vi "twoAxiesControl_Example.vi"() -> ()   [LabVIEW 2020]
uses:
  Recipe.vi
  ConnectionData.vi
  ConnectionData_Write.vi
  SMCD14_lib.lvlib
panel:
  in  "StopAppBtn":bool caption="Close"
  in  "Recipe":bool
  in  "Chart":bool
  in  "DisconnectBtn":bool
  in  "ConnectBtn":bool
  out "AxisControlSubPanelsArray":refnum<vi>[](array[refnum])
  in  "error in (no error)":errorcluster
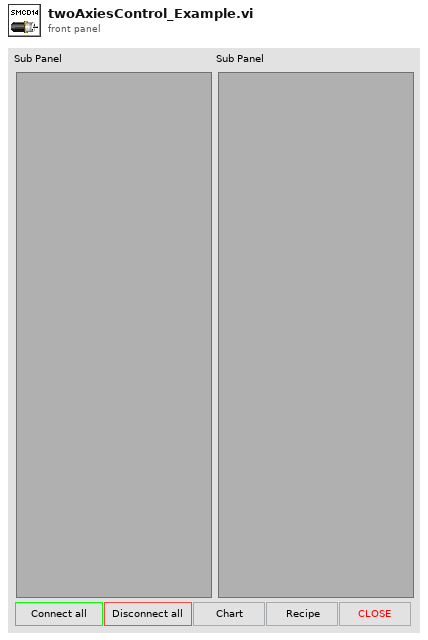
[diagram p1: front panel]
types:
  T1 = enum32{"Invalid", "Standard", "Closed", "Hidden", "Minimized", "Maximized"}
  T2 = enum32{"Bad", "Idle", "Run top level", "Running"}
  T3 = typedef "SMCD14_lib.lvlib/ConnectionData_typedef.ctl" = cluster{"DeviceIDCtrl":u16, "ProtocolCtrl":enum16{"Modbus RTU", "Modbus TCP", ""}, "COMportCtrl":refnum<visa-resource-name>, "IPCtrl":string, "serial master instance":refnum<class "Modbus Master.lvclass">, "ConnectionStatusIndicator":bool}
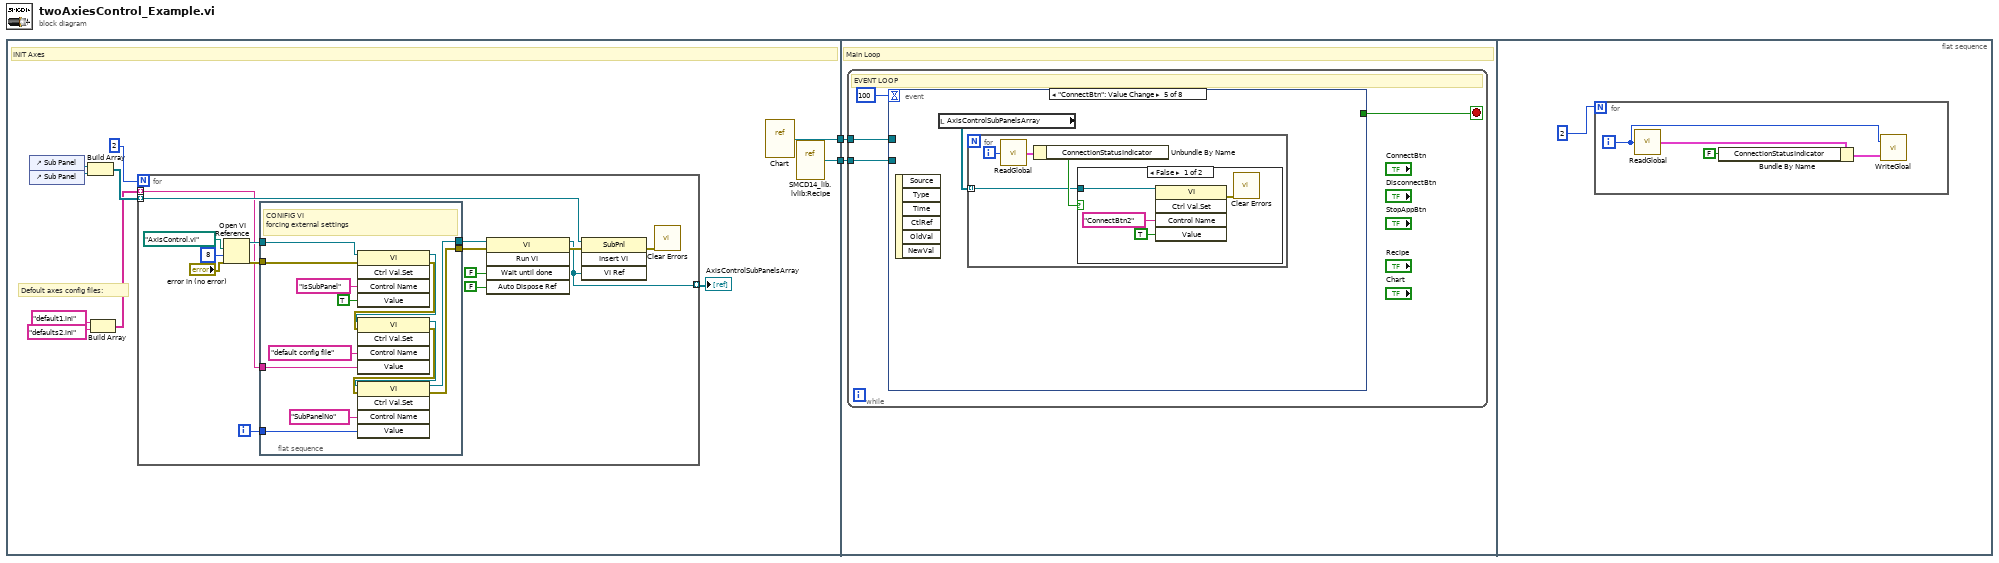
[diagram p0: block diagram]
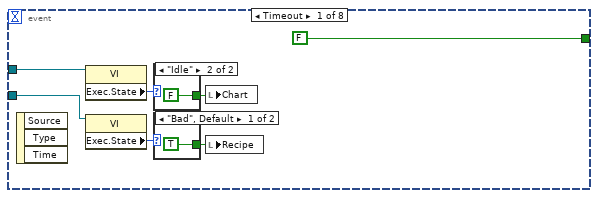
[diagram p2: hidden frame]
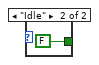
[diagram p3: hidden frame]
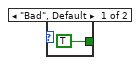
[diagram p4: hidden frame]
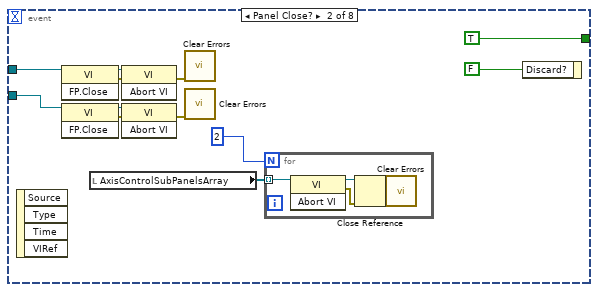
[diagram p5: hidden frame]
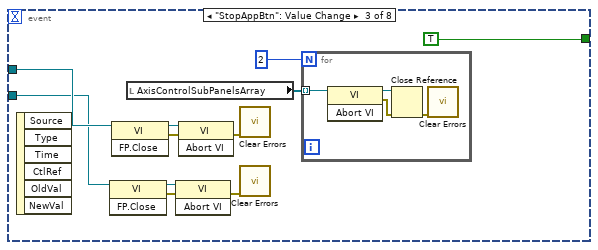
[diagram p6: hidden frame]
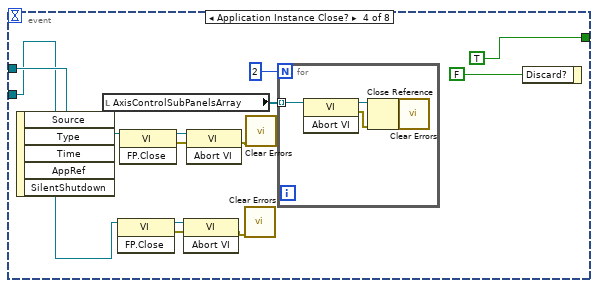
[diagram p7: hidden frame]
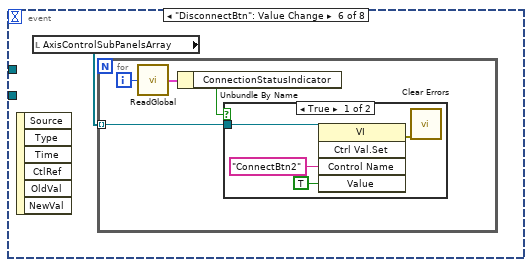
[diagram p9: hidden frame]
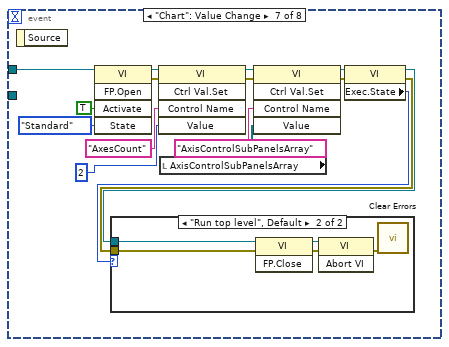
[diagram p11: hidden frame]
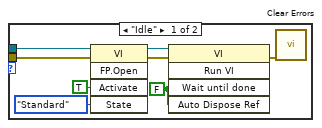
[diagram p12: hidden frame]
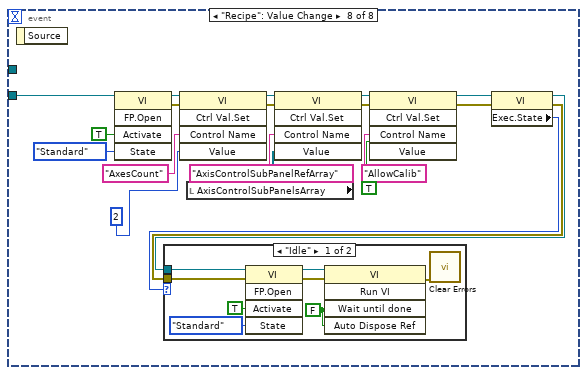
[diagram p13: hidden frame]
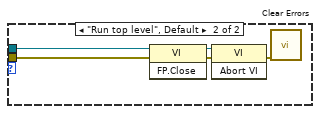
[diagram p14: hidden frame]
diagram:
  n1 = flat-sequence {
    tunnel: [w10] -> w2
    tunnel: [w9] -> w1
    tunnel: w2 -> [w43]
    tunnel: w1 -> [w42]
    frame #0 {
      # "Defoult axes config files:"
      # "INIT Axes"
      n2 = control-ref of="Sub Panel"() -> (w8:refnum<vi>)
      n3 = control-ref of="Sub Panel"() -> (w7:refnum<vi>)
      n4 = Build Array(w8, w7) -> (w11:refnum<vi>[])
      n5 = Build Array("default1.ini" ("default value"), "defaults2.ini" ("default value")) -> (w3:string[])
      n6 = for {
        N: 2 ("AxesCount") -> [_]
        tunnel: w11 -> [w24] mode=indexing
        tunnel: [w14] -> w12 mode=indexing
        tunnel: w3 -> [w16] mode=indexing
        i -> [w15]
        n7 = Open VI Reference(vi path=path "AxisControl.vi", options=8, error in (no error)="error in (no error)") -> (vi reference=w18:refnum<vi>, error out=w17:errorcluster)  [unwired: 3 in]
        n8 = flat-sequence {
          tunnel: w18 -> [w39]
          tunnel: [w30] -> w25
          tunnel: w17 -> [w38]
          tunnel: [w31] -> w23
          tunnel: w16 -> [w34]
          tunnel: w15 -> [w33]
          frame #0 {
            # "CONIFIG VI\nforcing external settings"
            n9 = invoke class="VI" method="Ctrl Val.Set"(reference=w39, error in=w38, "Control Name"="IsSubPanel", "Value"=TRUE) -> (reference out=w36:refnum<vi>, error out=w35:errorcluster)  [unwired: 1 in, 3 out]
            n10 = invoke class="VI" method="Ctrl Val.Set"(reference=w36, error in=w35, "Control Name"="default config file", "Value"=w34) -> (reference out=w29:refnum<vi>, error out=w28:errorcluster)  [unwired: 1 in, 3 out]
            n11 = invoke class="VI" method="Ctrl Val.Set"(reference=w29, error in=w28, "Control Name"="SubPanelNo", "Value"=w33) -> (reference out=w31:refnum<vi>, error out=w30:errorcluster)  [unwired: 1 in, 3 out]
          }
        }
        n12 = invoke class="VI" method="Run VI"(reference=w23, error in=w25, "Wait until done"=FALSE ("Wait Until Done"), "Auto Dispose Ref"=FALSE ("Auto Dispose Reference")) -> (reference out=w14:refnum<vi>, error out=w22:errorcluster)  [unwired: 1 in, 3 out]
        n13 = invoke class="SubPnl" method="Insert VI"(reference=w24, error in=w22, "VI Ref"=w14) -> (error out=w13:errorcluster)  [unwired: 1 in, 3 out]
        n14 = call <vilib>:"Clear Errors.vi"("error in (no error)"=w13) -> ()  [unwired: 5 in, 2 out]
      }
      "AxisControlSubPanelsArray" <- w12
      n15 = vi-ref "Chart.vi"() -> (w10:refnum<vi>)
      n16 = vi-ref "SMCD14_lib.lvlib:Recipe.vi"() -> (w9:refnum<vi>)
    }
    frame #1 {
      # "Main Loop"
      n17 = while {
        tunnel: w43 -> [w45]
        tunnel: w42 -> [w44]
        stop <- w46 stop-if-true
        # "EVENT LOOP"
        n18 = event shown="[4] \"ConnectBtn\": Value Change" {
          selector: _ -> [_ _ _ _ _ _ _ _]
          dyn-events: _ -> [_ _ _ _ _ _ _ _]
          timeout: 100 -> [_ _ _ _ _ _ _ _]
          tunnel: [FALSE ("Discard?") TRUE ("Discard?") TRUE ("Discard?") TRUE ("Discard?") _ _ _ _] -> w46
          tunnel: w45 -> [w53 w67 w83 w94 _ _ w134 _]
          tunnel: w44 -> [w49 w64 w80 w93 _ _ _ w161]
          event Timeout {
            n19 = event-data() -> ()  [unwired: 1 in, 3 out]
            n20 = property class="VI"(reference=w53) -> ("Exec.State"=w52:T2)  [unwired: 1 in, 2 out]
            n21 = property class="VI"(reference=w49) -> ("Exec.State"=w50:T2)  [unwired: 1 in, 2 out]
            n22 = case shown="\"Idle\"" w52 {
              tunnel: [TRUE ("Chart") FALSE ("Chart")] -> w51
              frame "Bad", Default {
              }
              frame "Idle" {
              }
            }
            n23 = case shown="\"Bad\", Default" w50 {
              tunnel: [TRUE ("Chart") FALSE ("Chart")] -> w48
              frame "Bad", Default {
              }
              frame "Idle" {
              }
            }
            n24 = local write "Chart"(w51) -> ()
            n25 = local write "Recipe"(w48) -> ()
          }
          event Panel Close? {
            n26 = event-data() -> ()  [unwired: 1 in, 4 out]
            n27 = invoke class="VI" method="FP.Close"(reference=w67) -> (reference out=w66:refnum<vi>, error out=w63:errorcluster)  [unwired: 2 in, 1 out]
            n28 = invoke class="VI" method="FP.Close"(reference=w64) -> (reference out=w65:refnum<vi>, error out=w62:errorcluster)  [unwired: 2 in, 1 out]
            n29 = local read "AxisControlSubPanelsArray"() -> (w70:refnum<vi>[])
            n30 = invoke class="VI" method="Abort VI"(reference=w66, error in=w63) -> (error out=w61:errorcluster)  [unwired: 1 in, 2 out]
            n31 = invoke class="VI" method="Abort VI"(reference=w65, error in=w62) -> (error out=w60:errorcluster)  [unwired: 1 in, 2 out]
            n32 = call <vilib>:"Clear Errors.vi"("error in (no error)"=w61) -> ()  [unwired: 5 in, 2 out]
            n33 = call <vilib>:"Clear Errors.vi"("error in (no error)"=w60) -> ()  [unwired: 5 in, 2 out]
            n34 = for {
              N: 2 ("AxesCount") -> [_]
              tunnel: w70 -> [w74] mode=indexing
              n35 = invoke class="VI" method="Abort VI"(reference=w74) -> (reference out=w73:refnum<vi>, error out=w72:errorcluster)  [unwired: 2 in, 1 out]
              n36 = Close Reference(reference=w73, error in (no error)=w72) -> (error out=w71:errorcluster)
              n37 = call <vilib>:"Clear Errors.vi"("error in (no error)"=w71) -> ()  [unwired: 5 in, 2 out]
            }
            n38 = event-data("Discard?"=FALSE) -> ()  [unwired: 1 in, 1 out]
          }
          event "StopAppBtn": Value Change {
            n39 = event-data() -> ()  [unwired: 1 in, 6 out]
            n40 = invoke class="VI" method="FP.Close"(reference=w80) -> (reference out=w81:refnum<vi>, error out=w78:errorcluster)  [unwired: 2 in, 1 out]
            n41 = invoke class="VI" method="FP.Close"(reference=w83) -> (reference out=w82:refnum<vi>, error out=w79:errorcluster)  [unwired: 2 in, 1 out]
            n42 = local read "AxisControlSubPanelsArray"() -> (w85:refnum<vi>[])
            n43 = invoke class="VI" method="Abort VI"(reference=w81, error in=w78) -> (error out=w77:errorcluster)  [unwired: 1 in, 2 out]
            n44 = invoke class="VI" method="Abort VI"(reference=w82, error in=w79) -> (error out=w76:errorcluster)  [unwired: 1 in, 2 out]
            n45 = call <vilib>:"Clear Errors.vi"("error in (no error)"=w76) -> ()  [unwired: 5 in, 2 out]
            n46 = call <vilib>:"Clear Errors.vi"("error in (no error)"=w77) -> ()  [unwired: 5 in, 2 out]
            n47 = for {
              N: 2 ("AxesCount") -> [_]
              tunnel: w85 -> [w89] mode=indexing
              n48 = invoke class="VI" method="Abort VI"(reference=w89) -> (reference out=w88:refnum<vi>, error out=w87:errorcluster)  [unwired: 2 in, 1 out]
              n49 = Close Reference(reference=w88, error in (no error)=w87) -> (error out=w86:errorcluster)
              n50 = call <vilib>:"Clear Errors.vi"("error in (no error)"=w86) -> ()  [unwired: 5 in, 2 out]
            }
          }
          event Application Instance Close? {
            n51 = event-data() -> ()  [unwired: 1 in, 5 out]
            n52 = local read "AxisControlSubPanelsArray"() -> (w96:refnum<vi>[])
            n53 = invoke class="VI" method="FP.Close"(reference=w93) -> (reference out=w98:refnum<vi>, error out=w100:errorcluster)  [unwired: 2 in, 1 out]
            n54 = invoke class="VI" method="FP.Close"(reference=w94) -> (reference out=w97:refnum<vi>, error out=w99:errorcluster)  [unwired: 2 in, 1 out]
            n55 = invoke class="VI" method="Abort VI"(reference=w98, error in=w100) -> (error out=w91:errorcluster)  [unwired: 1 in, 2 out]
            n56 = invoke class="VI" method="Abort VI"(reference=w97, error in=w99) -> (error out=w92:errorcluster)  [unwired: 1 in, 2 out]
            n57 = call <vilib>:"Clear Errors.vi"("error in (no error)"=w91) -> ()  [unwired: 5 in, 2 out]
            n58 = call <vilib>:"Clear Errors.vi"("error in (no error)"=w92) -> ()  [unwired: 5 in, 2 out]
            n59 = for {
              N: 2 ("AxesCount") -> [_]
              tunnel: w96 -> [w105] mode=indexing
              n60 = invoke class="VI" method="Abort VI"(reference=w105) -> (reference out=w104:refnum<vi>, error out=w103:errorcluster)  [unwired: 2 in, 1 out]
              n61 = Close Reference(reference=w104, error in (no error)=w103) -> (error out=w102:errorcluster)
              n62 = call <vilib>:"Clear Errors.vi"("error in (no error)"=w102) -> ()  [unwired: 5 in, 2 out]
            }
            n63 = event-data("Discard?"=FALSE) -> ()  [unwired: 1 in, 1 out]
          }
          event "ConnectBtn": Value Change {
            n64 = event-data() -> ()  [unwired: 1 in, 6 out]
            n65 = local read "AxisControlSubPanelsArray"() -> (w106:refnum<vi>[])
            n66 = for {
              tunnel: w106 -> [w107] mode=indexing
              i -> [w109]
              n67 = call-poly "ReadGlobal.vi"("AxisNo"=w109) -> ("ConnectionDataOUT"=w110:T3)
              n68 = Unbundle By Name(w110) -> ("ConnectionStatusIndicator"=w108:bool)
              n69 = case shown="False" w108 {
                tunnel: w107 -> [w112 _]
                frame False {
                  n70 = invoke class="VI" method="Ctrl Val.Set"(reference=w112, "Control Name"="ConnectBtn2", "Value"=TRUE) -> (error out=w111:errorcluster)  [unwired: 2 in, 4 out]
                  n71 = call <vilib>:"Clear Errors.vi"("error in (no error)"=w111) -> ()  [unwired: 5 in, 2 out]
                }
                frame True {
                }
              }
            }
          }
          event "DisconnectBtn": Value Change {
            n72 = event-data() -> ()  [unwired: 1 in, 6 out]
            n73 = local read "AxisControlSubPanelsArray"() -> (w115:refnum<vi>[])
            n74 = for {
              tunnel: w115 -> [w116] mode=indexing
              i -> [w118]
              n75 = call-poly "ReadGlobal.vi"("AxisNo"=w118) -> ("ConnectionDataOUT"=w119:T3)
              n76 = Unbundle By Name(w119) -> ("ConnectionStatusIndicator"=w117:bool)
              n77 = case shown="True" w117 {
                tunnel: w116 -> [w121 _]
                frame True {
                  n78 = invoke class="VI" method="Ctrl Val.Set"(reference=w121, "Control Name"="ConnectBtn2", "Value"=TRUE) -> (error out=w120:errorcluster)  [unwired: 2 in, 4 out]
                  n79 = call <vilib>:"Clear Errors.vi"("error in (no error)"=w120) -> ()  [unwired: 5 in, 2 out]
                }
                frame False {
                }
              }
            }
          }
          event "Chart": Value Change {
            n80 = event-data() -> ()  [unwired: 1 in, 1 out]
            n81 = invoke class="VI" method="FP.Open"(reference=w134, "Activate"=TRUE ("Activate?"), "State"=T1."Standard") -> (reference out=w138:refnum<vi>, error out=w137:errorcluster)  [unwired: 2 in, 3 out]
            n82 = invoke class="VI" method="Ctrl Val.Set"(reference=w138, error in=w137, "Control Name"="AxesCount", "Value"=2 ("AxesCount")) -> (reference out=w129:refnum<vi>, error out=w128:errorcluster)  [unwired: 1 in, 3 out]
            n83 = local read "AxisControlSubPanelsArray"() -> (w130:refnum<vi>[])
            n84 = invoke class="VI" method="Ctrl Val.Set"(reference=w129, error in=w128, "Control Name"="AxisControlSubPanelsArray", "Value"=w130) -> (reference out=w127:refnum<vi>, error out=w126:errorcluster)  [unwired: 1 in, 3 out]
            n85 = property class="VI"(reference=w127, error in=w126) -> (reference out=w133:refnum<vi>, error out=w132:errorcluster, "Exec.State"=w125:T2)
            n86 = case shown="\"Run top level\", Default" w125 {
              tunnel: w133 -> [w141 w152]
              tunnel: w132 -> [w140 w151]
              frame "Idle" {
                w147 = FALSE ("Activate?")
                n87 = invoke class="VI" method="FP.Open"(reference=w141, error in=w140, "Activate"=TRUE ("Activate?"), "State"=T1."Standard") -> (reference out=w145:refnum<vi>, error out=w146:errorcluster)  [unwired: 1 in, 3 out]
                n88 = invoke class="VI" method="Run VI"(reference=w145, error in=w146, "Wait until done"=w147, "Auto Dispose Ref"=w147) -> (error out=w142:errorcluster)  [unwired: 1 in, 4 out]
                n89 = call <vilib>:"Clear Errors.vi"("error in (no error)"=w142) -> ()  [unwired: 5 in, 2 out]
              }
              frame "Run top level", Default {
                n90 = invoke class="VI" method="FP.Close"(reference=w152, error in=w151) -> (reference out=w150:refnum<vi>, error out=w149:errorcluster)  [unwired: 1 in, 1 out]
                n91 = invoke class="VI" method="Abort VI"(reference=w150, error in=w149) -> (error out=w148:errorcluster)  [unwired: 1 in, 2 out]
                n92 = call <vilib>:"Clear Errors.vi"("error in (no error)"=w148) -> ()  [unwired: 5 in, 2 out]
              }
            }
          }
          event "Recipe": Value Change {
            n93 = event-data() -> ()  [unwired: 1 in, 1 out]
            n94 = invoke class="VI" method="FP.Open"(reference=w161, "Activate"=TRUE ("Activate?"), "State"=T1."Standard") -> (reference out=w172:refnum<vi>, error out=w171:errorcluster)  [unwired: 2 in, 3 out]
            n95 = invoke class="VI" method="Ctrl Val.Set"(reference=w172, error in=w171, "Control Name"="AxesCount", "Value"=2 ("AxesCount")) -> (reference out=w163:refnum<vi>, error out=w162:errorcluster)  [unwired: 1 in, 3 out]
            n96 = local read "AxisControlSubPanelsArray"() -> (w164:refnum<vi>[])
            n97 = invoke class="VI" method="Ctrl Val.Set"(reference=w163, error in=w162, "Control Name"="AxisControlSubPanelRefArray", "Value"=w164) -> (reference out=w159:refnum<vi>, error out=w158:errorcluster)  [unwired: 1 in, 3 out]
            n98 = invoke class="VI" method="Ctrl Val.Set"(reference=w159, error in=w158, "Control Name"="AllowCalib", "Value"=TRUE) -> (reference out=w157:refnum<vi>, error out=w156:errorcluster)  [unwired: 1 in, 3 out]
            n99 = property class="VI"(reference=w157, error in=w156) -> (reference out=w168:refnum<vi>, error out=w166:errorcluster, "Exec.State"=w167:T2)
            n100 = case shown="\"Idle\"" w167 {
              tunnel: w168 -> [w175 w185]
              tunnel: w166 -> [w174 w184]
              frame "Idle" {
                w180 = FALSE ("Activate?")
                n101 = invoke class="VI" method="FP.Open"(reference=w175, error in=w174, "Activate"=TRUE ("Activate?"), "State"=T1."Standard") -> (reference out=w178:refnum<vi>, error out=w179:errorcluster)  [unwired: 1 in, 3 out]
                n102 = invoke class="VI" method="Run VI"(reference=w178, error in=w179, "Wait until done"=w180, "Auto Dispose Ref"=w180) -> (error out=w173:errorcluster)  [unwired: 1 in, 4 out]
                n103 = call <vilib>:"Clear Errors.vi"("error in (no error)"=w173) -> ()  [unwired: 5 in, 2 out]
              }
              frame "Run top level", Default {
                n104 = invoke class="VI" method="FP.Close"(reference=w185, error in=w184) -> (reference out=w183:refnum<vi>, error out=w182:errorcluster)  [unwired: 1 in, 1 out]
                n105 = invoke class="VI" method="Abort VI"(reference=w183, error in=w182) -> (error out=w181:errorcluster)  [unwired: 1 in, 2 out]
                n106 = call <vilib>:"Clear Errors.vi"("error in (no error)"=w181) -> ()  [unwired: 5 in, 2 out]
              }
            }
          }
        }
      }
    }
    frame #2 {
      n107 = for {
        N: 2 ("AxesCount") -> [_]
        i -> [w187]
        n108 = call-poly "ReadGlobal.vi"("AxisNo"=w187) -> ("ConnectionDataOUT"=w190:T3)
        n109 = Bundle By Name(cluster=w190, "ConnectionStatusIndicator"=FALSE) -> (w189:T3)
        n110 = call-poly "WriteGloal.vi"("ConnectionDataIN"=w189, "AxisNo"=w187) -> ()  [unwired: 1 in]
      }
    }
  }
